vi "Jacobian.vi"() -> ()   [LabVIEW 2024]
uses:
  ME121-25-main/ME121-25-main/LabVIEW/SerialVIs/subs/portX.xctl
  <vilib>/Analysis/baseanly.llb/A x Vector.vi
  <vilib>/Analysis/baseanly.llb/Real Inverse Matrix.vi
  <vilib>/Analysis/NI_AALBase.lvlib
panel:
  out "concatenated string":string
  out "Q1":dbl
  out "Q2":dbl
  in  "portX 2":refnum<visa-resource-name>(xcontrol)="ASRL10"
  in  "geometry":cluster{"L 1":dbl, "L 2":dbl, "q":dbl[]}={"L 1"=77.5, "L 2"=85.0, "q"=[20.0, 100.0]}
  out "end effector":cluster{"X":dbl, "Y":dbl}={"X"=20.22785471594338, "Y"=-59.70688630406909}
  out "2D Picture":picture
  out "end (2D)":cluster{"x":dbl, "y":dbl}={"x"=120.22785471594338, "y"=159.7068863040691}
  in  "picture in":picture
  in  "stop":bool
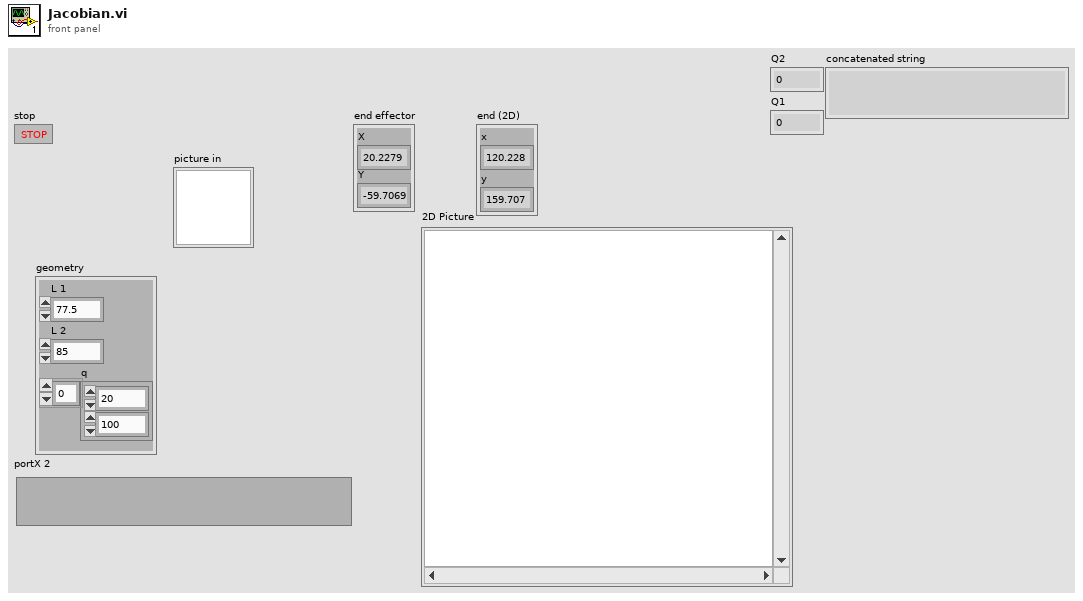
[diagram p1: front panel]
types:
  T1 = typedef "NI_Matrix.lvlib/RealMatrix.ctl" = dbl[][]
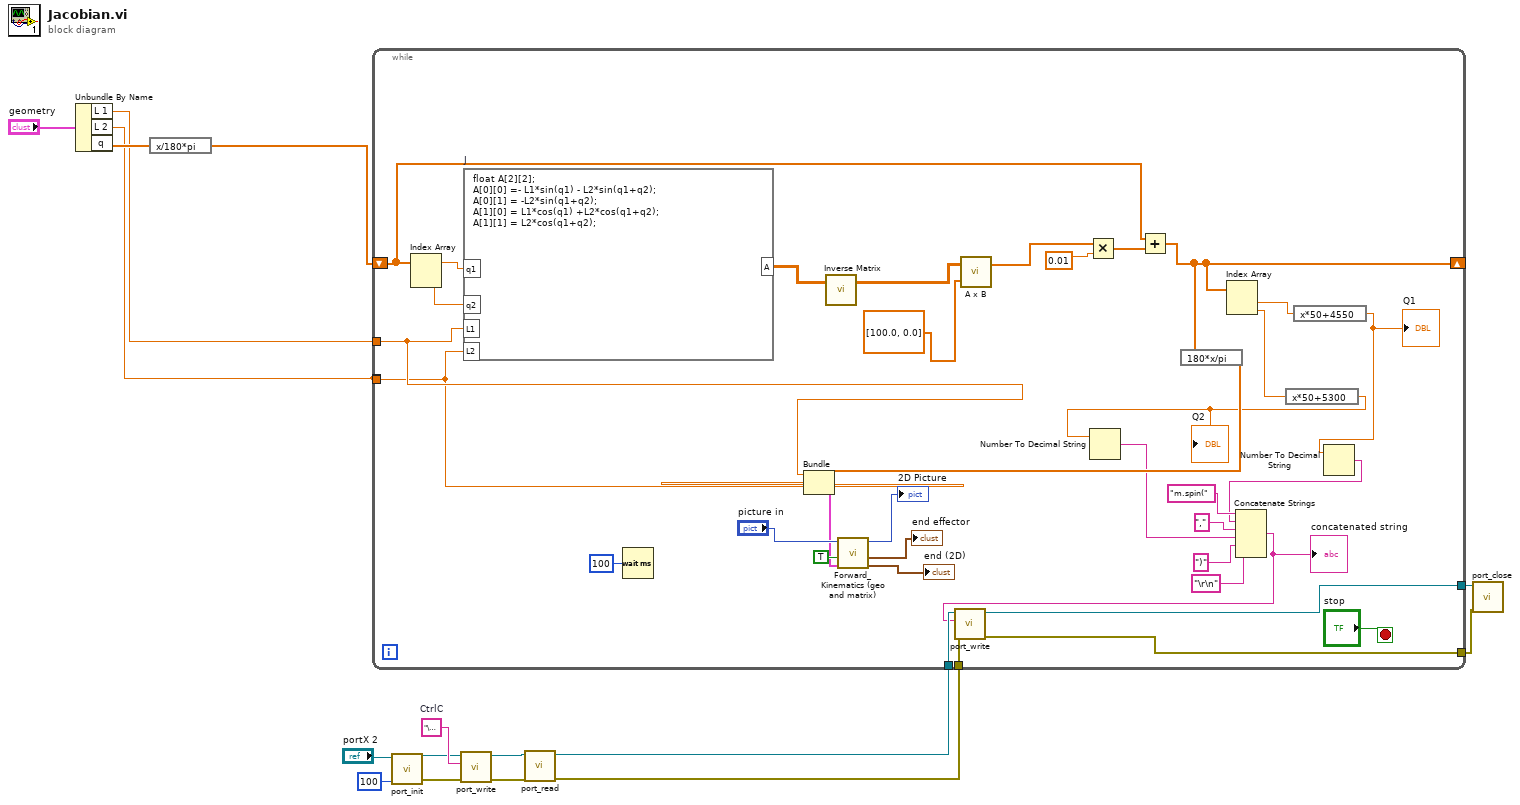
[diagram p0: block diagram]
diagram:
  w11 = "\u0003"  # CtrlC
  n1 = Unbundle By Name "Unbundle By Name"("geometry") -> ("L 1"=w15:dbl, "L 2"=w14:dbl, "q"=w16:dbl[])
  n2 = expression code="x/180*pi"(w16) -> (w12:dbl[])
  n3 = call "port_init.vi"("Timeout (ms)"=u32 100, "VISA Refnum in"="portX 2") -> ("error out"=w9:errorcluster, "VISA Refnum out"=w10:refnum<visa-resource-name>)  [unwired: 8 in]
  n4 = call "port_write.vi"("error in (no error)"=w9, "write buffer"=w11, "VISA Refnum in"=w10) -> ("error out"=w7:errorcluster, "VISA Refnum out"=w8:refnum<visa-resource-name>)  [unwired: 7 in]
  n5 = call "port_read.vi"("error in (no error)"=w7, "VISA Refnum in"=w8) -> ("error out"=w1:errorcluster, "VISA Refnum out"=w2:refnum<visa-resource-name>)  [unwired: 7 in, 1 out]
  n6 = while {
    shift-right: [w24] -> _
    shift-left: w12 -> [w48]
    tunnel: w15 -> [w41]
    tunnel: w14 -> [_]
    tunnel: w14 -> [w40]
    tunnel: [w32] -> w4
    tunnel: [w31] -> w3
    tunnel: w2 -> [w30]
    tunnel: w1 -> [w29]
    stop <- "stop" stop-if-true
    n7 = Index Array(array=w48) -> (element #1=w36:dbl, element #2=w35:dbl)  [unwired: 2 in]
    n8 = formula code="float A[2][2];\nA[0][0] =- L1*sin(q1) - L2*sin(q1+q2);\nA[0][1] = -L2*sin(q1+q2);\nA[1][0] = L1*cos(q1) +L2*cos(q1+q2);\nA[1][1] = L2*cos(q1+q2);" "J"("q1"=w36, "q2"=w35, "L1"=w41, "L2"=w40) -> ("A"=w52:dbl[][])
    n9 = Wait (ms)(milliseconds to wait=u32 100) -> ()  [unwired: 1 out]
    n10 = call-poly <vilib>:"Inverse Matrix.vi"("Input Matrix"=w52) -> ("Inverse Matrix"=w51:T1)  [unwired: 1 in, 1 out]
    n11 = call-poly <vilib>:"A x B.vi"("Vector"=dbl[] [100.0, 0.0], "A"=w51) -> ("A x Vector"=w37:dbl[])  [unwired: 1 out]
    n12 = Multiply(x=w37, y=0.01) -> (x*y=w47:dbl[])
    n13 = Add(x=w48, y=w47) -> (x+y=w24:dbl[])
    n14 = expression code="180*x/pi"(w24) -> (w34:dbl[])
    n15 = Bundle("L 1"=w41, "L 2"=w40, w34) -> (w33:cluster{"L 1":dbl, "L 2":dbl, dbl[]})  [unwired: 1 in]
    n16 = call "Forward_Kinematics (geo and matrix).vi"("geometry"=w33, "geometry?"=TRUE, "picture in"="picture in") -> ("end (2D)"=→"end (2D)":cluster{"x":dbl, "y":dbl}, "end effector"=→"end effector":cluster{"X":dbl, "Y":dbl}, "2D Picture"=→"2D Picture":picture)  [unwired: 6 in]
    n17 = Index Array(array=w24) -> (element #1=w23:dbl, element #2=w22:dbl)  [unwired: 2 in]
    n18 = expression code="x*50+5300"(w22) -> (w21:dbl)
    "Q2" <- w21
    n19 = Number To Decimal String(number=w21) -> (decimal integer string=w19:string)  [unwired: 1 in]
    n20 = expression code="x*50+4550"(w23) -> (w17:dbl)
    "Q1" <- w17
    n21 = Number To Decimal String(number=w17) -> (decimal integer string=w20:string)  [unwired: 1 in]
    n22 = Concatenate Strings("m.spin(" ("string"), w20, "," ("string"), w19, ")" ("string"), "\r\n" ("string")) -> (w18:string)
    "concatenated string" <- w18
    n23 = call "port_write.vi"("error in (no error)"=w29, "write buffer"=w18, "VISA Refnum in"=w30) -> ("error out"=w31:errorcluster, "VISA Refnum out"=w32:refnum<visa-resource-name>)  [unwired: 7 in]
  }
  n24 = call "port_close.vi"("error in (no error)"=w3, "VISA Refnum in"=w4) -> ()  [unwired: 10 in]
